vi "cmc-function-gen.vi"() -> ()   [LabVIEW 2010]
panel:
  out "XY Graph":cluster{"Y":dbl[], "Y":dbl[]}[](graph)
  out "f(x) Array":dbl[](array[numeric])
  out "x Array":dbl[](array[numeric])
  in  "# of divisions":u32
  in  "end x = 'b'":dbl
  in  "Start x = 'a'":dbl
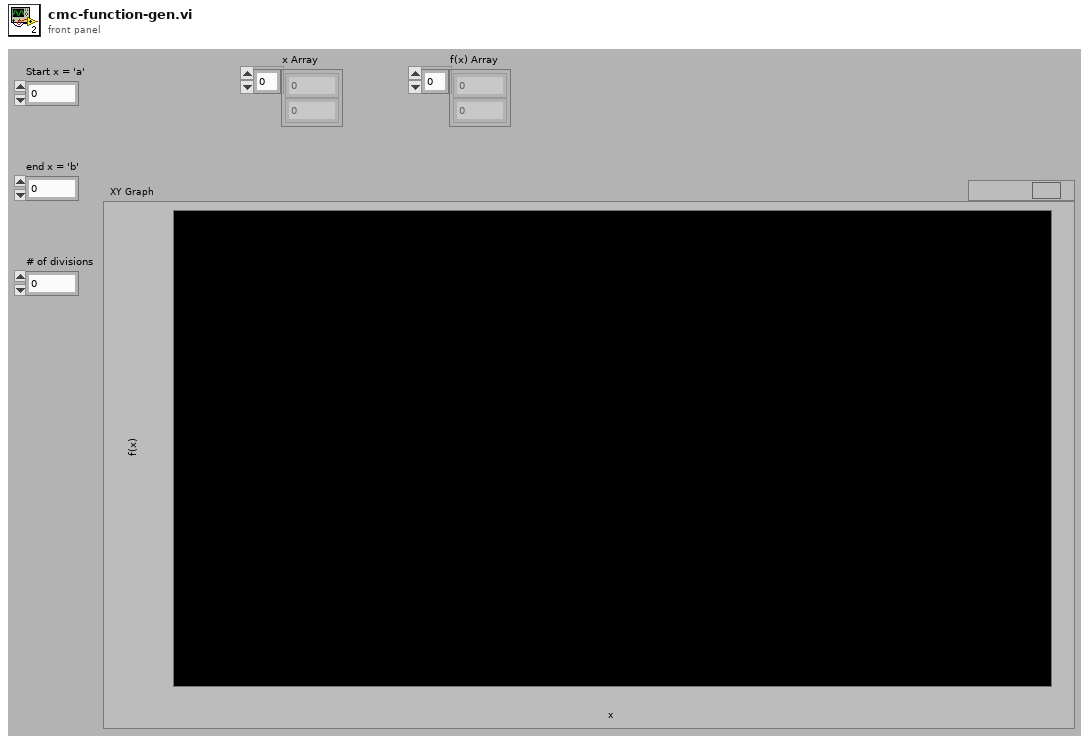
[diagram p1: front panel]
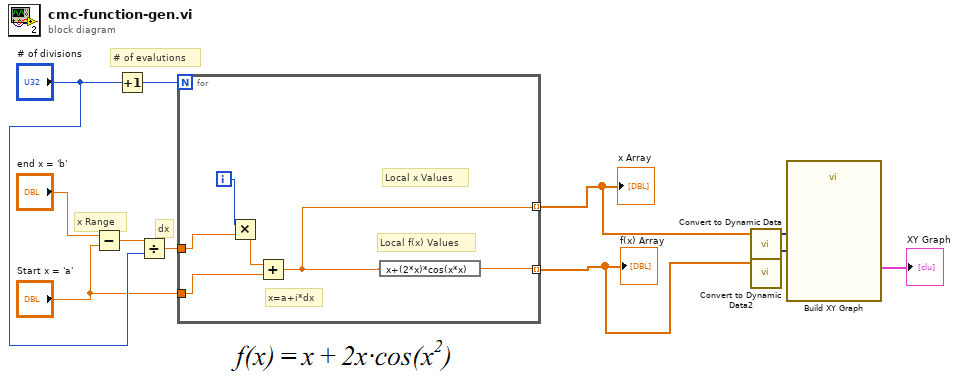
[diagram p0: block diagram]
diagram:
  # "dx"
  # "x Range"
  # "# of evalutions"
  n1 = Subtract(x="end x = 'b'", y="Start x = 'a'") -> (x-y=w10:dbl)
  n2 = Increment(x="# of divisions") -> (x+1=w11:u32)
  n3 = Divide(x=w10, y="# of divisions") -> (x/y=w8:dbl)
  n4 = for {
    N: w11 -> [_]
    tunnel: w8 -> [w16]
    tunnel: "Start x = 'a'" -> [w15]
    tunnel: [w13] -> w4 mode=indexing
    tunnel: [w12] -> w2 mode=indexing
    i -> [w17]
    # "Local f(x) Values"
    # "x=a+i*dx"
    # "Local x Values"
    n5 = Multiply(x=w17, y=w16) -> (x*y=w14:dbl)
    n6 = Add(x=w14, y=w15) -> (x+y=w13:dbl)
    n7 = expression code="x+(2*x)*cos(x*x)"(w13) -> (w12:dbl)
  }
  "x Array" <- w4
  "f(x) Array" <- w2
  n8 = call "Convert to Dynamic Data"("Array"=w4) -> ("Dynamic Data Type"=w3:dynamicdata)  [unwired: 3 in]
  n9 = call "Convert to Dynamic Data2"("Array"=w2) -> ("Dynamic Data Type"=w1:dynamicdata)  [unwired: 3 in]
  n10 = call "Build XY Graph"("Y Input"=w1, "X Input"=w3) -> ("XY Graph"=→"XY Graph":cluster{"Y":dbl[], "Y":dbl[]}[])  [unwired: 3 in, 6 out]
